vi "Configure PID Kp.vi"(8 "error in (no error)":errorcluster, 9 "PID Kp":sgl, 10 "node address (same)":u8, 11 "ProPar in":refnum<class "PL Bronkhorst ProPar.lvclass">) -> (0 "error out":errorcluster, 3 "ProPar out":refnum<class "PL Bronkhorst ProPar.lvclass">)   [LabVIEW 2015, in "PL Bronkhorst ProPar.lvclass"]
doc: "Configures PID controller proportional term of the specified <b>node</b>."
uses:
  PL Bronkhorst ProPar.lvclass
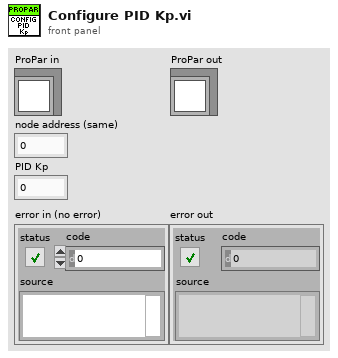
[diagram p1: front panel]
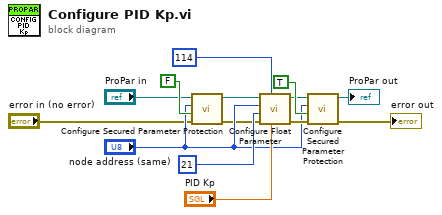
[diagram p0: block diagram]
diagram:
  n1 = call "Configure Secured Parameter Protection.vi"("error in (no error)"="error in (no error)", "enable protection"=FALSE, "node"="node address (same)", "ProPar in"="ProPar in") -> ("error out"=w2:errorcluster, "ProPar out"=w3:refnum<class "PL Bronkhorst ProPar.lvclass">)  [unwired: 6 in]
  n2 = call "Configure Float Parameter.vi"("value"="PID Kp", "process number"=u8 114, "error in (no error)"=w2, "parameter number"=u8 21 ("process number"), "node"="node address (same)", "ProPar in"=w3) -> ("error out"=w7:errorcluster, "ProPar out"=w8:refnum<class "PL Bronkhorst ProPar.lvclass">)  [unwired: 4 in]
  n3 = call "Configure Secured Parameter Protection.vi"("error in (no error)"=w7, "enable protection"=TRUE, "node"="node address (same)", "ProPar in"=w8) -> ("error out"=→"error out":errorcluster, "ProPar out"=→"ProPar out":refnum<class "PL Bronkhorst ProPar.lvclass">)  [unwired: 6 in]
